vi "Graph.vi"() -> ()   [LabVIEW 2017]
panel:
  out "appended array":dbl[](array[numeric])
  in  "stop 2":bool
  out "Waveform Chart 2":waveform(dbl)[](graph)
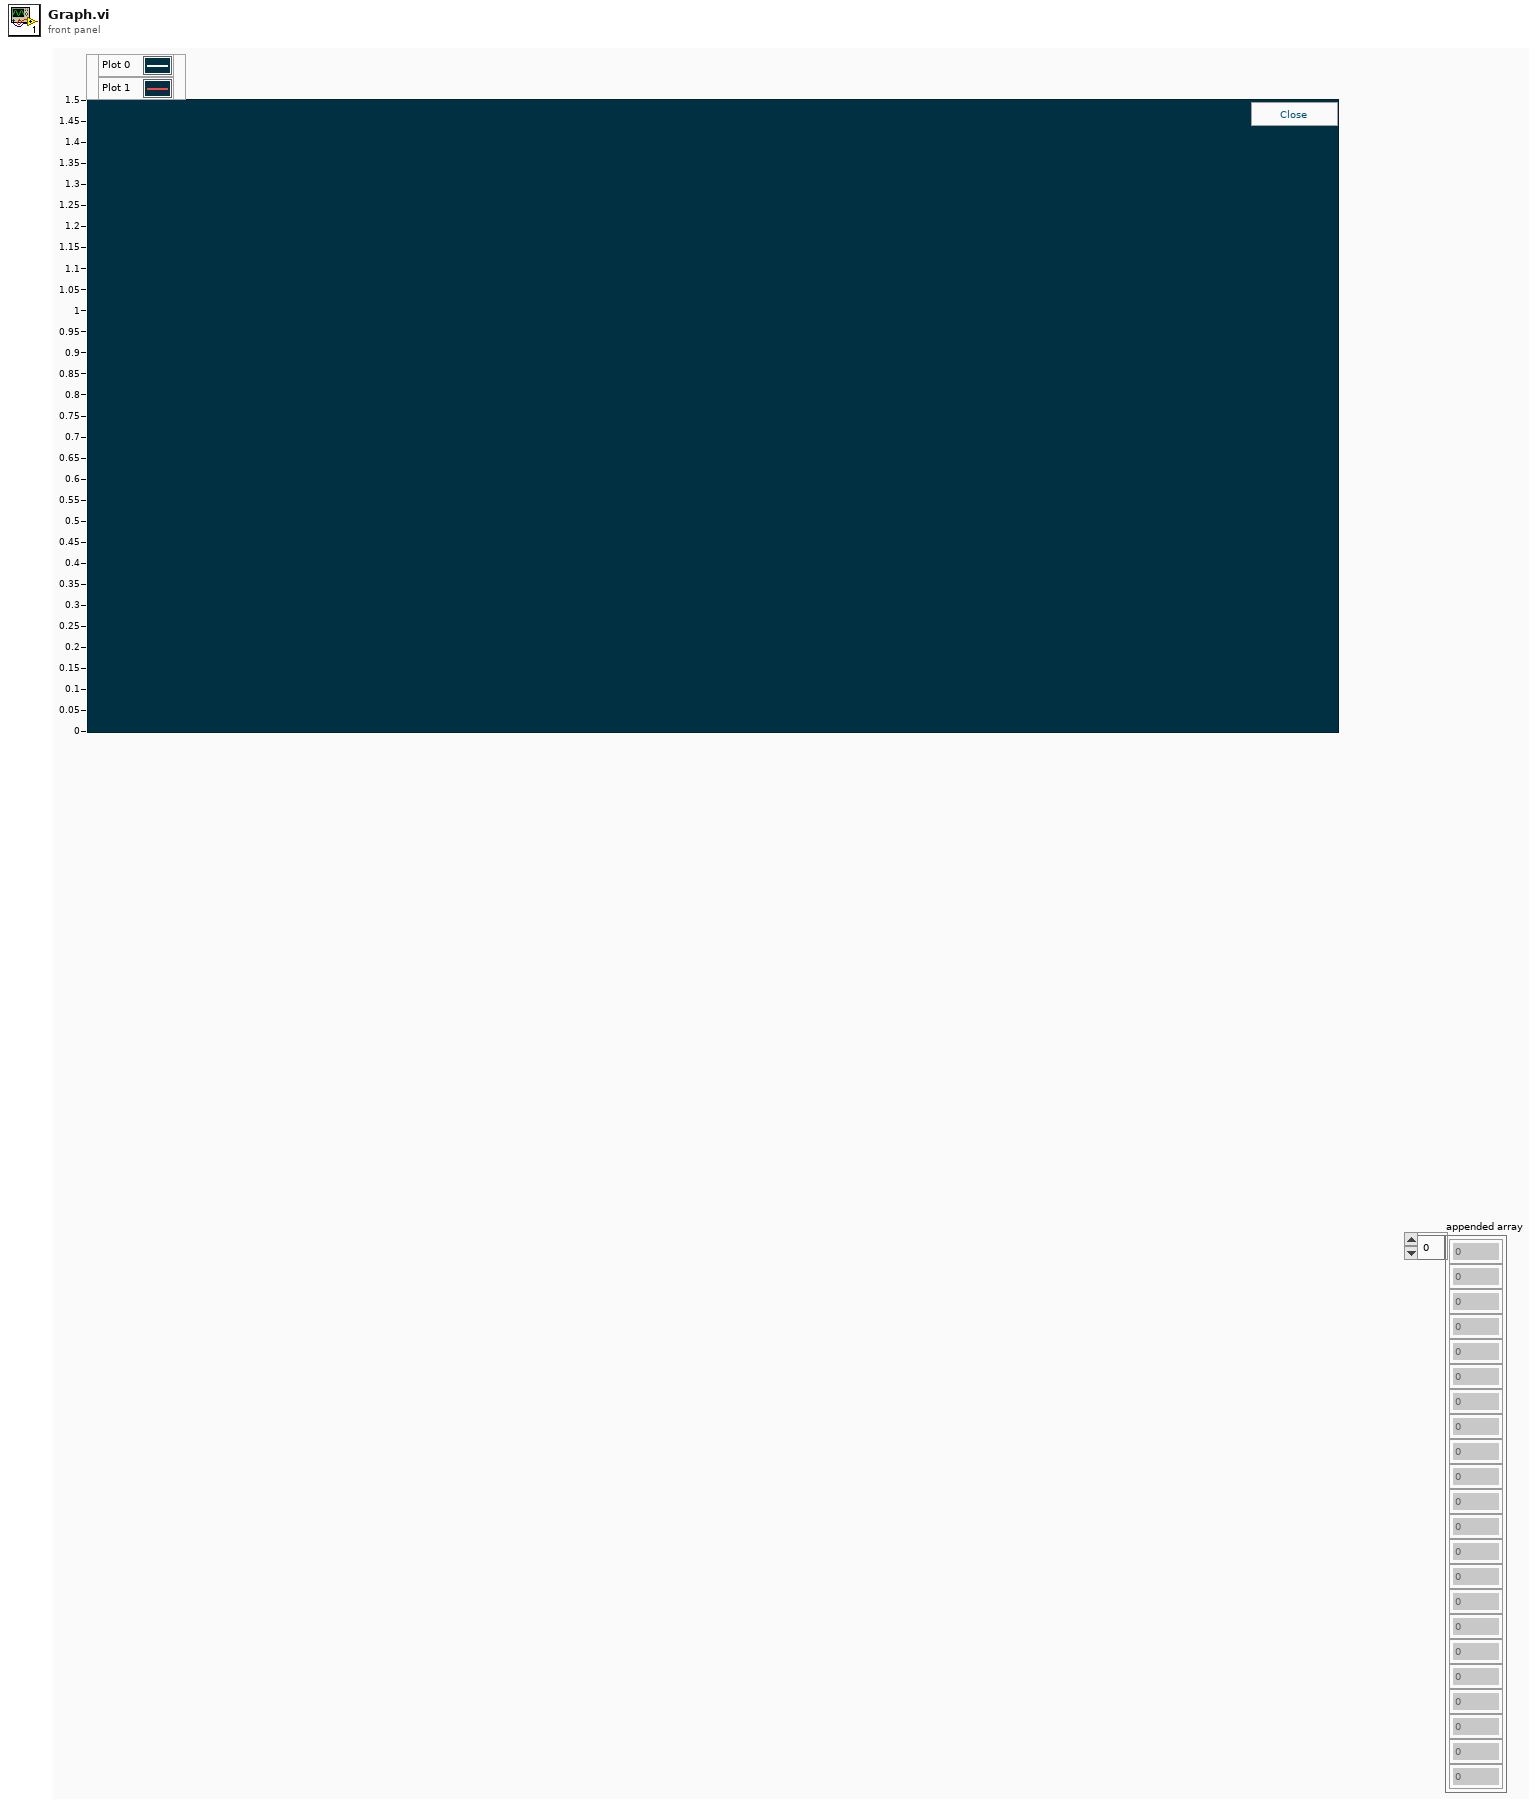
[diagram p1: front panel]
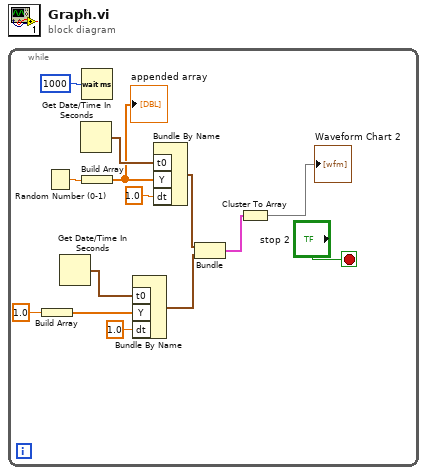
[diagram p0: block diagram]
diagram:
  n1 = while {
    stop <- "stop 2" stop-if-true
    n2 = Build Array(1.0 ("element")) -> (w5:dbl[])
    n3 = Random Number (0-1)() -> (number: 0 to 1=w12:dbl)
    n4 = Get Date/Time In Seconds() -> (seconds since 1Jan1904=w6:timestamp)
    n5 = Get Date/Time In Seconds() -> (seconds since 1Jan1904=w14:timestamp)
    n6 = Wait (ms)(milliseconds to wait=u32 1000 ("millisecond multiple")) -> ()  [unwired: 1 out]
    n7 = Build Array(w12) -> (w13:dbl[])
    "appended array" <- w13
    n8 = Bundle By Name("t0"=w6, "Y"=w5, "dt"=1.0) -> (w3:waveform(dbl))  [unwired: 1 in]
    n9 = Bundle By Name("t0"=w14, "Y"=w13, "dt"=1.0) -> (w7:waveform(dbl))  [unwired: 1 in]
    n10 = Bundle(w7, w3) -> (w2:cluster{waveform(dbl), waveform(dbl)})  [unwired: 1 in]
    n11 = Cluster To Array(cluster=w2) -> (array=→"Waveform Chart 2":waveform(dbl)[])
  }
